vi "Game Sim (SubVI).vi"(9 "Reset":bool, 10 "Jump":bool) -> (1 "Fail":bool, 2 "Score":i32, 3 "Picture":i32[][](graph))   [LabVIEW 2013]
doc: "Simulates the Flappy Bird game."
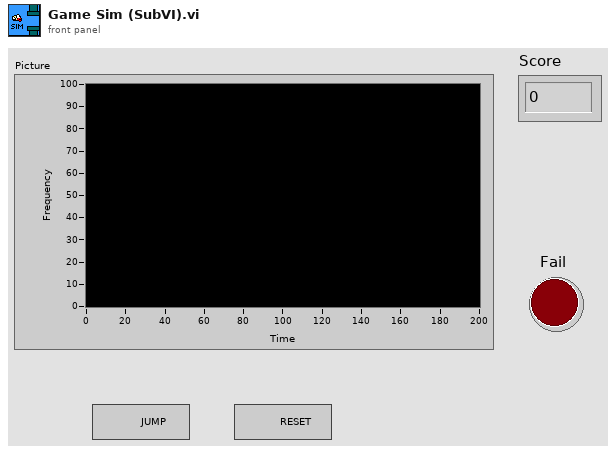
[diagram p1: front panel]
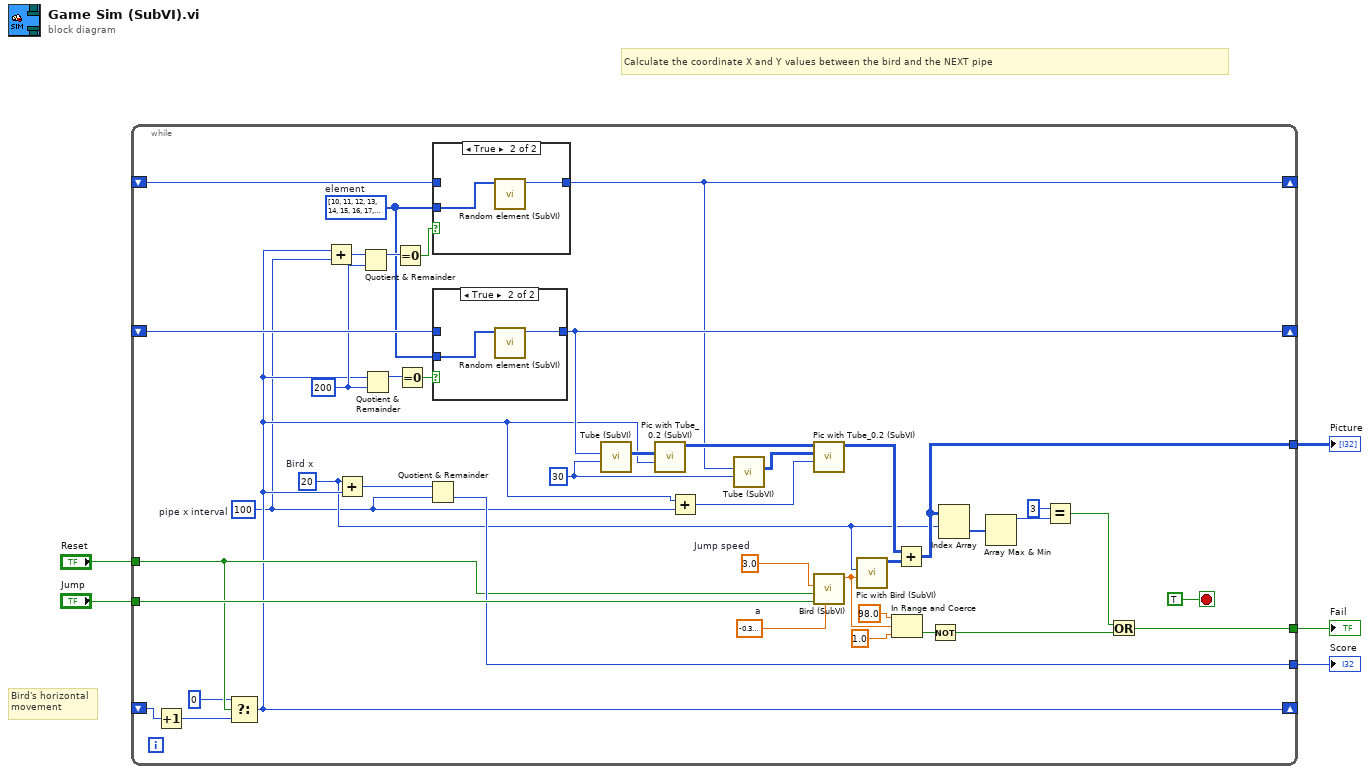
[diagram p0: block diagram]
diagram:
  # "Calculate the coordinate X and Y values between the bird and the NEXT pipe"
  # "Bird's horizontal\nmovement"
  n1 = while {
    shift-right: [w30] -> _
    shift-left: _ -> [w31]
    shift-right: [w24] -> _
    shift-left: _ -> [w25]
    tunnel: "Jump" -> [w16]
    tunnel: [w15] -> w4
    tunnel: [w14] -> w3
    tunnel: [w13] -> w2
    tunnel: "Reset" -> [w12]
    shift-right: [w8] -> _
    shift-left: _ -> [w10]
    stop <- TRUE stop-if-true
    w18 = i32[] [10, 11, 12, 13, 14, 15, 16, 17, 18, 19, 20, 21, 22, 23, 24, 25, 26, 27, 28, 29, 30, 31, 32, 33, 34, 35, 36, 37, 38, 39, 40, 41, 42, 43, 44, 45, 46, 47, 48, 49, 50, 51, 52, 53, 54, 55, 56, 57, 58, 59]  # element
    w23 = -0.30000000000000004  # a
    w46 = 3.0  # Jump speed
    w7 = 20  # Bird x
    w6 = 100  # pipe x interval
    w27 = 200 ("y")
    w43 = 30 ("Gap height (30)")
    n2 = Increment(x=w10) -> (x+1=w9:i32)
    n3 = Select(t=0, s=w12, f=w9) -> (s? t:f=w8:i32)
    n4 = Add(x=w8, y=w6) -> (x+y=w28:i32)
    n5 = Add(x=w7, y=w8) -> (x+y=w19:i32)
    n6 = Quotient & Remainder(x=w28, y=w27) -> (x-y*floor(x/y)=w29:i32)  [unwired: 1 out]
    n7 = Quotient & Remainder(x=w8, y=w27) -> (x-y*floor(x/y)=w33:i32)  [unwired: 1 out]
    n8 = Equal To 0?(x=w29) -> (x = 0?=w26:bool)
    n9 = Equal To 0?(x=w33) -> (x = 0?=w32:bool)
    n10 = Quotient & Remainder(x=w19, y=w6) -> (floor(x/y)=w13:i32)  [unwired: 1 out]
    n11 = case shown="True" w26 {
      tunnel: [w48 w50] -> w24
      tunnel: w25 -> [w48 _]
      tunnel: w18 -> [_ w49]
      frame False {
      }
      frame True {
        n12 = call "Random element (SubVI).vi"("Array"=w49) -> ("random element"=w50:i32)  [unwired: 10 in]
      }
    }
    n13 = case shown="True" w32 {
      tunnel: [w51 w53] -> w30
      tunnel: w31 -> [w51 _]
      tunnel: w18 -> [_ w52]
      frame False {
      }
      frame True {
        n14 = call "Random element (SubVI).vi"("Array"=w52) -> ("random element"=w53:i32)  [unwired: 10 in]
      }
    }
    n15 = call "Tube (SubVI).vi"("Gap height (30)"=w43, "Gap low y"=w30) -> ("Tube"=w45:i32[][])  [unwired: 9 in]
    n16 = call "Pic with Tube_0.2 (SubVI).vi"("Tube x"=w8, "Tube"=w45) -> ("Picture"=w44:i32[][])  [unwired: 9 in]
    n17 = Add(x=w8, y=w6) -> (x+y=w20:i32)
    n18 = call "Tube (SubVI).vi"("Gap height (30)"=w43, "Gap low y"=w24) -> ("Tube"=w22:i32[][])  [unwired: 9 in]
    n19 = call "Pic with Tube_0.2 (SubVI).vi"("Tube x"=w20, "Tube"=w22, "Picture in"=w44) -> ("Picture"=w21:i32[][])  [unwired: 8 in]
    n20 = call "Bird (SubVI).vi"("a"=w23, "Jump"=w16, "Reset"=w12, "Jump speed"=w46) -> ("Position"=w42:dbl)  [unwired: 7 in]
    n21 = call "Pic with Bird (SubVI).vi"("Bird Position"=w42, "X position"=w7) -> ("Picture"=w47:i32[][])  [unwired: 9 in]
    n22 = In Range and Coerce(upper limit=98.0, x=w42, lower limit=1.0) -> (In Range?=w39:bool)  [unwired: 1 out]
    n23 = Add(x=w21, y=w47) -> (x+y=w15:i32[][])
    n24 = Not(x=w39) -> (.not. x?=w35:bool)
    n25 = Index Array(array=w15, index (row)=w7) -> (element=w38:i32[])  [unwired: 1 in]
    n26 = Array Max & Min(array=w38) -> (max value=w37:i32)  [unwired: 3 out]
    n27 = Equal?(x=3 ("y"), y=w37) -> (x = y?=w34:bool)
    n28 = Or(x=w34, y=w35) -> (x .or. y?=w14:bool)
  }
  "Picture" <- w4
  "Fail" <- w3
  "Score" <- w2
